vi "Set Channel Values Block Data Ref.vi"(8 "error in":errorcluster, 9 "Values Array in":dbl[](array[numeric]), 10 "Block Data Ref":T1[](array[typedef]) {"Data Reference" format="%.0x"}, 11 "VS Engine in":refnum<class "VS Engine.lvclass">) -> (0 "error out":errorcluster, 1 "Values Array out":dbl[](array[numeric]), 2 "Block Data Ref dup":T1[](array[typedef]) {"Data Reference" format="%.0x"}, 3 "VS Engine out":refnum<class "VS Engine.lvclass">)   [LabVIEW 2024, in "VS Engine Abstraction.lvlib" / "VS Engine.lvclass"]
uses:
  VS Engine.lvclass
  VS Engine.lvclass/VS Engine.ctl
  <vilib>/NI VeriStand/Custom Device API/Custom Device API.lvlib
  <vilib>/NI VeriStand/Custom Device API/Data Reference.ctl
  <vilib>/NI VeriStand/Custom Device API/Block Data Reference.ctl
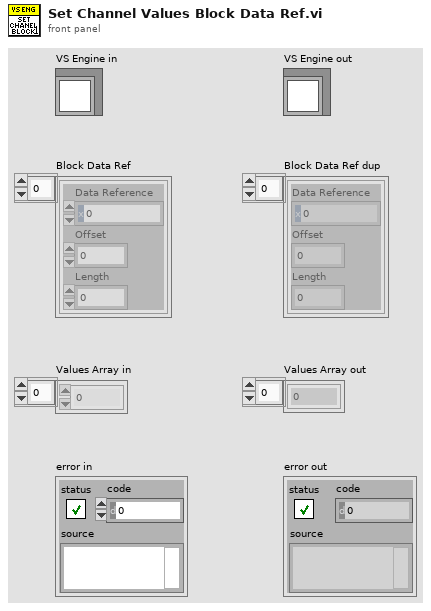
[diagram p1: front panel]
types:
  T1 = typedef "Custom Device API.lvlib/Block Data Reference.ctl" = cluster{"Data Reference":T2, "Offset":u64, "Length":u64}
  T2 = typedef "Custom Device API.lvlib/Data Reference.ctl" = i32
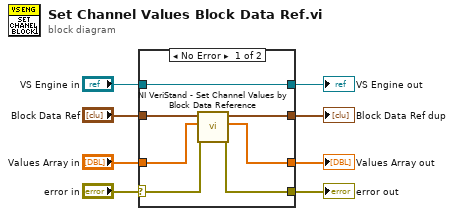
[diagram p0: block diagram]
diagram:
  n1 = case shown="No Error" "error in" {
    selector: "error in" -> [w15 w19]
    tunnel: [w14 w19] -> w7
    tunnel: [w13 w18] -> w5
    tunnel: "VS Engine in" -> [w13 w18]
    tunnel: "Block Data Ref" -> [w12 w17]
    tunnel: "Values Array in" -> [w11 w16]
    tunnel: [w10 w17] -> w2
    tunnel: [w9 w16] -> w1
    frame No Error {
      n2 = call <vilib>:"NI VeriStand - Set Channel Values by Block Data Reference.vi"("error in (no error)"=w15, "Values Array in"=w11, "Block Data Ref"=w12) -> ("error out"=w14:errorcluster, "Values Array out"=w9:dbl[], "Block Data Ref dup"=w10:T1[])  [unwired: 6 in]
    }
    frame Error {
    }
  }
  "error out" <- w7
  "VS Engine out" <- w5
  "Values Array out" <- w1
  "Block Data Ref dup" <- w2
